vi "execute.vi"(8 "error in (no error)":errorcluster, 9 "DataCollection in (B)":refnum<class "GenericComponent.lvclass">, 10 "ImagingMode in (A)":refnum<class "GenericComponent.lvclass">, 11 "AdapterMH110616ImagingModeToDataCollection in":refnum<class "AdapterMH110616ImagingModeToDataCollection.lvclass">) -> (0 "error out":errorcluster, 1 "DataCollection out (B)":refnum<class "GenericComponent.lvclass">, 2 "ImagingMode out (A)":refnum<class "GenericComponent.lvclass">, 3 "AdapterMH110616ImagingModeToDataCollection out":refnum<class "AdapterMH110616ImagingModeToDataCollection.lvclass">)   [LabVIEW 2010, in "AdapterMH110616ImagingModeToDataCollection.lvclass"]
uses:
  AdapterMH110616ImagingModeToDataCollection.lvclass
  common/classes/GenericComponent/GenericComponent/GenericComponent.lvclass
  ImagingMode/ImagingModeDL090130Frame/ImagingModeDL090130Frame/ImagingModeDL090130Frame.lvclass
  DataCollection/DataCollectionDL090215/DataCollectionDL090215/DataCollectionDL090215.lvclass
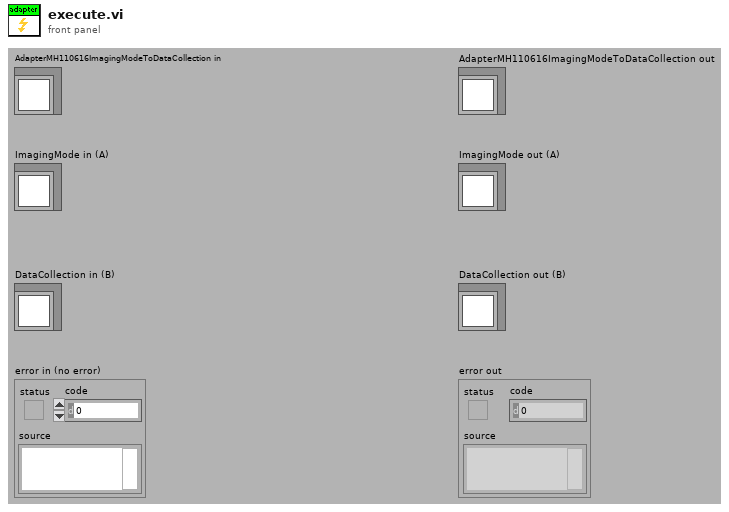
[diagram p1: front panel]
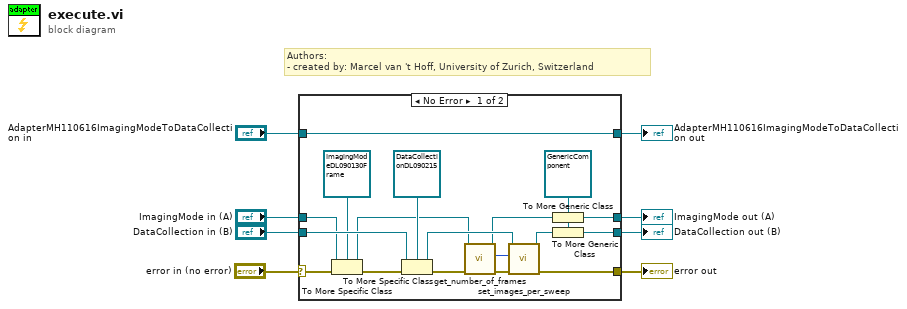
[diagram p0: block diagram]
diagram:
  # "Authors: \n- created by: Marcel van 't Hoff, University of Zurich, Switzerland"
  n1 = case shown="No Error" "error in (no error)" {
    selector: "error in (no error)" -> [w23 w29]
    tunnel: [w19 w29] -> w7
    tunnel: [w26 w30] -> w6
    tunnel: "AdapterMH110616ImagingModeToDataCollection in" -> [w26 w30]
    tunnel: "DataCollection in (B)" -> [w25 w27]
    tunnel: "ImagingMode in (A)" -> [w24 w28]
    tunnel: [w16 w27] -> w2
    tunnel: [w15 w28] -> w1
    frame No Error {
      w20 = refnum<class "GenericComponent.lvclass"> refnum ("GenericComponent.lvclass")
      n2 = To More Specific Class(target class=refnum<class "ImagingModeDL090130Frame.lvclass"> refnum ("ImagingModeDL090130Frame.lvclass"), reference=w24, error in=w23) -> (specific class reference=w13:refnum<class "ImagingModeDL090130Frame.lvclass">, error out=w22:errorcluster)
      n3 = To More Specific Class(target class=refnum<class "DataCollectionDL090215.lvclass"> refnum ("DataCollectionDL090215.lvclass"), reference=w25, error in=w22) -> (specific class reference=w18:refnum<class "DataCollectionDL090215.lvclass">, error out=w10:errorcluster)
      n4 = call-dynamic "get_number_of_frames.vi"("error in (no error)"=w10, "ImagingModeDL090130Frame in"=w13) -> ("error out"=w9:errorcluster, "number of frames"=w11:i32, "ImagingModeDL090130Frame out"=w12:refnum<class "ImagingModeDL090130Frame.lvclass">)  [unwired: 7 in]
      n5 = call-dynamic "set_images_per_sweep.vi"("error in (no error)"=w9, "images per sweep"=w11, "DL090215DataCollection.lvclass in"=w18) -> ("error out"=w19:errorcluster, "DL090215DataCollection.lvclass out"=w17:refnum<class "DataCollectionDL090215.lvclass">)  [unwired: 7 in]
      n6 = To More Generic Class(target class=w20, reference=w12) -> (generic class reference=w15:refnum<class "GenericComponent.lvclass">)
      n7 = To More Generic Class(target class=w20, reference=w17) -> (generic class reference=w16:refnum<class "GenericComponent.lvclass">)
    }
    frame Error {
    }
  }
  "error out" <- w7
  "AdapterMH110616ImagingModeToDataCollection out" <- w6
  "ImagingMode out (A)" <- w1
  "DataCollection out (B)" <- w2
